vi "GetHDF5TreeItemIcons.vi"(6 "error in (no error)":errorcluster, 7 "Object Types":T1[](array[typedef]) items=["H5G_UNKNOWN"=-1, "H5G_GROUP"=0, "H5G_DATASET"=1, "H5G_TYPE"=2, "H5G_LINK"=3, "H5G_UDLINK"=4], 8 "Object Names":string[](array[string]), 9 "HDF5 Loc Ref":T3) -> (0 "error out":errorcluster, 1 "Object Types out":T1[](array[typedef]) items=["H5G_UNKNOWN"=-1, "H5G_GROUP"=0, "H5G_DATASET"=1, "H5G_TYPE"=2, "H5G_LINK"=3, "H5G_UDLINK"=4], 2 "Object Names out":string[](array[string]), 3 "HDF5 Loc Ref out":T3, 4 "Item Icons":T2[](array[typedef]))   [LabVIEW 2017]
uses:
  <vilib>/UPVI/lvhdf5/group.llb/H5G_obj_t.ctl
  <vilib>/UPVI/lvhdf5/library.llb/HDF5 Ref.ctl
  <vilib>/UPVI/lvhdf5/utility.llb/private/TreeIconsEnum.ctl
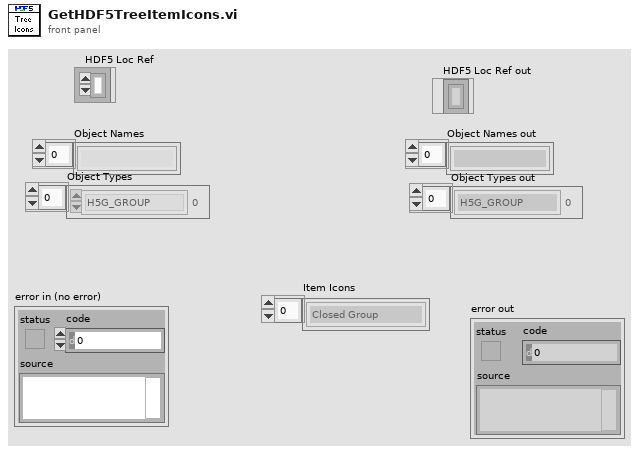
[diagram p1: front panel]
types:
  T1 = typedef "H5G_obj_t.ctl" = i32
  T2 = typedef "TreeIconsEnum.ctl" = enum16{"None", "Closed Group", "Open Group", "Array Dataset", "Compound Dataset", "Datatype"}
  T3 = typedef "HDF5 Ref.ctl" = refnum<k1>
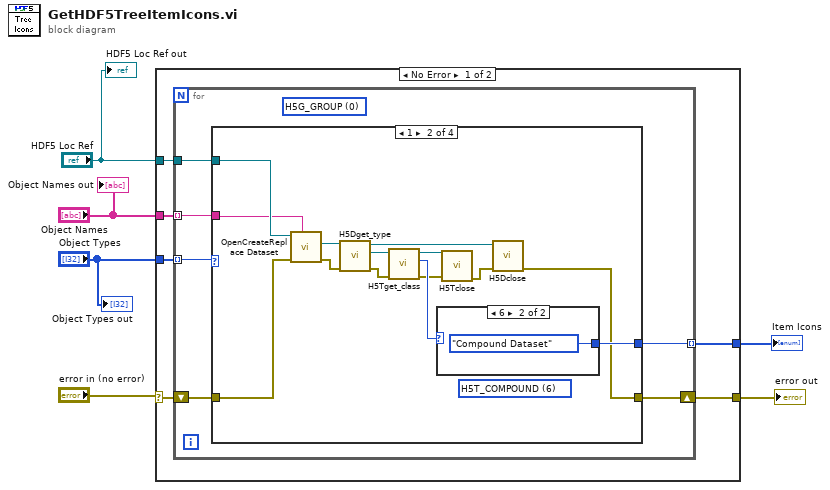
[diagram p0: block diagram]
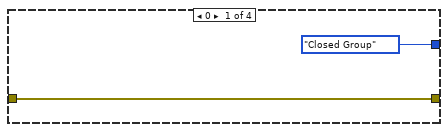
[diagram p2: hidden frame]
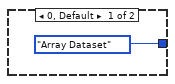
[diagram p3: hidden frame]
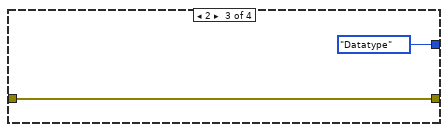
[diagram p4: hidden frame]
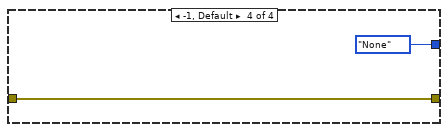
[diagram p5: hidden frame]
diagram:
  n1 = case shown="No Error" "error in (no error)" {
    selector: "error in (no error)" -> [w8 w41]
    tunnel: "HDF5 Loc Ref" -> [w10 _]
    tunnel: "Object Names" -> [w11 _]
    tunnel: "Object Types" -> [w12 _]
    tunnel: [w9 w41] -> w5
    tunnel: [w7 _] -> w4
    frame No Error {
      n2 = for {
        tunnel: w12 -> [w18] mode=indexing
        tunnel: w11 -> [w17] mode=indexing
        tunnel: w10 -> [w16]
        shift-right: [w13] -> w9
        shift-left: w8 -> [w15]
        tunnel: [w14] -> w7 mode=indexing
        (unwired) T1 0 items=["H5G_UNKNOWN"=-1, "H5G_GROUP"=0, "H5G_DATASET"=1, "H5G_TYPE"=2, "H5G_LINK"=3, "H5G_UDLINK"=4] ("Object Type")
        n3 = case shown="1" w18 {
          tunnel: w17 -> [_ w33 _ _]
          tunnel: w16 -> [_ w34 _ _]
          tunnel: w15 -> [w20 w32 w37 w39]
          tunnel: [TreeIconsEnum."Closed Group" ("TreeIcons") w26 TreeIconsEnum."Datatype" ("TreeIcons") TreeIconsEnum."None" ("TreeIcons")] -> w14
          tunnel: [w20 w21 w37 w39] -> w13
          frame 0 {
          }
          frame 1 {
            (unwired) 6 items=["H5T_NO_CLASS"=-1, "H5T_INTEGER"=0, "H5T_FLOAT"=1, "H5T_TIME"=2, "H5T_STRING"=3, "H5T_BITFIELD"=4, "H5T_OPAQUE"=5, "H5T_COMPOUND"=6, "H5T_REFERENCE"=7, "H5T_ENUM"=8, "H5T_VLEN"=9, "H5T_ARRAY"=10] ("class")
            n4 = call <vilib>:"OpenCreateReplace Dataset.vi"("Dataset Path"=w33, "error in (no error)"=w32, "HDF5 Ref"=w34) -> ("error out"=w31:errorcluster, "HDF5 Dataset Ref"=w30:T3)  [unwired: 6 in, 1 out]
            n5 = call <vilib>:"H5Dget_type.vi"("error in (no error)"=w31, "HDF5 Dataset Ref"=w30) -> ("error out"=w29:errorcluster, "HDF5 Datatype Ref"=w28:T3, "HDF5 Dataset Ref out"=w22:T3)  [unwired: 5 in]
            n6 = call <vilib>:"H5Tget_class.vi"("error in (no error)"=w29, "HDF5 Type Ref"=w28) -> ("error out"=w25:errorcluster, "class"=w27:i32, "HDF5 Type Ref out"=w24:T3)  [unwired: 5 in]
            n7 = case shown="6" w27 {
              tunnel: [TreeIconsEnum."Array Dataset" ("TreeIcons") TreeIconsEnum."Compound Dataset" ("TreeIcons")] -> w26
              frame 0, Default {
              }
              frame 6 {
              }
            }
            n8 = call <vilib>:"H5Tclose.vi"("error in (no error)"=w25, "HDF5 Datatype Ref"=w24) -> ("error out"=w23:errorcluster)  [unwired: 7 in]
            n9 = call <vilib>:"H5Dclose.vi"("error in (no error)"=w23, "HDF5 Dataset Ref"=w22) -> ("error out"=w21:errorcluster)  [unwired: 7 in]
          }
          frame 2 {
          }
          frame -1, Default {
          }
        }
      }
    }
    frame Error {
    }
  }
  "error out" <- w5
  "Item Icons" <- w4
  "HDF5 Loc Ref out" <- "HDF5 Loc Ref"
  "Object Names out" <- "Object Names"
  "Object Types out" <- "Object Types"
